vi "GOOP_AddCtrlToVIIfNeeded.vi"(11 "Ctrl VI in":refnum<vi>) -> (3 "VI out":refnum<vi>)   [LabVIEW 2012]
uses:
  <vilib>/Utility/miscctls.llb/LVPointTypeDef.ctl
panel:
  out "error out":errorcluster
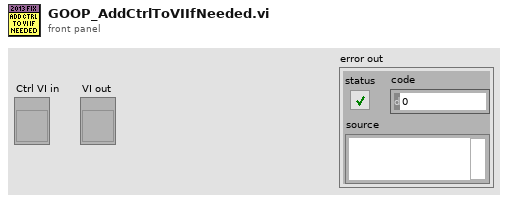
[diagram p1: front panel]
types:
  T1 = typedef "LVPointTypeDef.ctl" = cluster{"Horizontal":i16, "Vertical":i16}
  T2 = enum32{"invalid VI type", "Standard VI", "Control VI", "Global VI", "Polymorphic VI", "Configuration VI", "SubSystem", "Facade VI", "Method VI", "Statechart Diagram VI"}
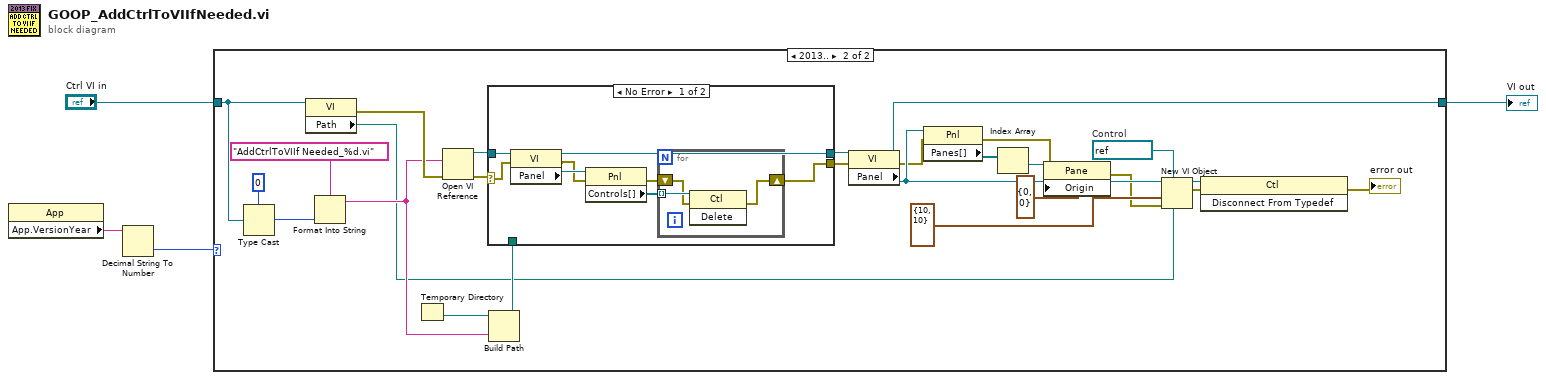
[diagram p0: block diagram]
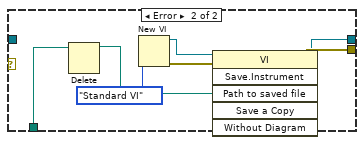
[diagram p3: hidden frame]
diagram:
  n1 = property class="App"() -> ("App.VersionYear"=w4:string)  [unwired: 2 in, 2 out]
  n2 = Decimal String To Number(string=w4) -> (number=w3:i32)  [unwired: 2 in, 1 out]
  n3 = case shown="2013.." w3 {
    tunnel: "Ctrl VI in" -> [w5 w14]
    tunnel: [w5 w19] -> w1
    frame Default {
    }
    frame 2013.. {
      w18 = refnum<vi> refnum  # Control
      n4 = Type Cast(type=u32 0, x=w14) -> (*(type *) &x=w13:u32)
      n5 = property class="VI"(reference=w14) -> (error out=w30:errorcluster, "Path"=w9:path)  [unwired: 1 in, 1 out]
      n6 = Format Into String(format string="AddCtrlToVIIf Needed_%d.vi", w13) -> (resulting string=w11:string)  [unwired: 2 in, 1 out]
      n7 = Temporary Directory() -> (w31:path)
      n8 = Open VI Reference(vi path=w11, error in (no error)=w30) -> (vi reference=w28:refnum<vi>, error out=w29:errorcluster)  [unwired: 4 in]
      n9 = Build Path(base path=w31, name or relative path=w11) -> (appended path=w27:path)
      n10 = case shown="No Error" w29 {
        selector: w29 -> [w34 _]
        tunnel: w28 -> [w39 _]
        tunnel: w27 -> [_ w49]
        tunnel: [w33 w44] -> w26
        tunnel: [w32 w46] -> w17
        frame No Error {
          n11 = property class="VI"(reference=w39, error in=w34) -> (reference out=w33:refnum<vi>, error out=w35:errorcluster, "Panel"=w38:refnum<vi>)
          n12 = property class="Pnl"(reference=w38, error in=w35) -> (error out=w36:errorcluster, "Controls[]"=w37:refnum<vi>[])  [unwired: 1 out]
          n13 = for {
            tunnel: w37 -> [w42] mode=indexing
            shift-right: [w40] -> w32
            shift-left: w36 -> [w41]
            n14 = invoke class="Ctl" method="Delete"(reference=w42, error in=w41) -> (error out=w40:errorcluster)  [unwired: 1 in, 2 out]
          }
        }
        frame Error {
          n15 = Delete(path (use dialog)=w49) -> (deleted path=w43:path)  [unwired: 4 in, 2 out]
          n16 = New VI(9:T2."Standard VI" ("vi type (standard vi)")) -> (0:w48:errorcluster, 3:w45:refnum<vi>)  [unwired: 6 in]
          n17 = invoke class="VI" method="Save.Instrument"(reference=w45, error in=w48, "Path to saved file"=w43) -> (reference out=w44:refnum<vi>, error out=w46:errorcluster)  [unwired: 3 in, 4 out]
        }
      }
      n18 = property class="VI"(reference=w26, error in=w17) -> (reference out=w19:refnum<vi>, error out=w16:errorcluster, "Panel"=w24:refnum<vi>)
      n19 = property class="Pnl"(reference=w24, error in=w16) -> (error out=w15:errorcluster, "Panes[]"=w23:refnum<vi>[])  [unwired: 1 out]
      n20 = Index Array(array=w23) -> (element=w22:refnum<vi>)  [unwired: 1 in]
      n21 = property class="Pane"(reference=w22, error in=w15, "Origin"=T1 {"Horizontal"=0, "Vertical"=0}) -> (error out=w20:errorcluster)  [unwired: 1 out]
      n22 = New VI Object(vi object class=w18, owner refnum=w24, position/next to=T1 {"Horizontal"=10, "Vertical"=10} ("location"), 6:w9, 8:w20) -> (object refnum=w8:refnum<vi>, 0:w6:errorcluster)  [unwired: 3 in]
      n23 = invoke class="Ctl" method="Disconnect From Typedef"(reference=w8, error in=w6) -> (error out=→"error out":errorcluster)  [unwired: 1 in, 2 out]
    }
  }
  "VI out" <- w1
